vi "Logic Calculator.vi"() -> ()   [LabVIEW 2016]
panel:
  out "Loops":i32
  in  "stop":bool
  out "not(x or y)?":bool
  out "not(x and y)?":bool
  out "x or y?":bool
  out "x and y?":bool
  in  "Boolean 2":bool
  in  "Boolean":bool
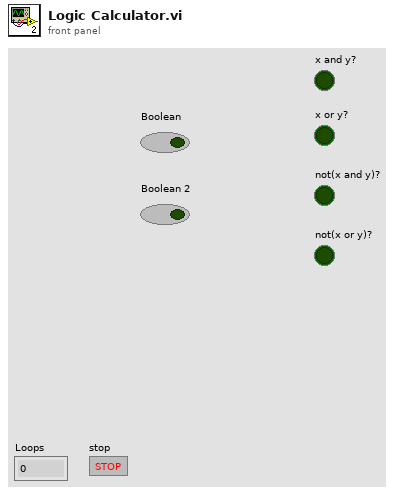
[diagram p1: front panel]
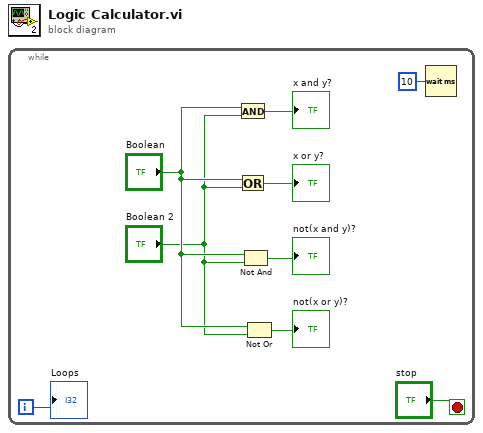
[diagram p0: block diagram]
diagram:
  n1 = while {
    i -> [w2]
    stop <- "stop" stop-if-true
    n2 = And(x="Boolean", y="Boolean 2") -> (x .and. y?=→"x and y?":bool)
    n3 = Or(x="Boolean", y="Boolean 2") -> (x .or. y?=→"x or y?":bool)
    n4 = Not And(1:"Boolean 2", 2:"Boolean") -> (0:→"not(x and y)?":bool)
    n5 = Not Or(1:"Boolean 2", 2:"Boolean") -> (0:→"not(x or y)?":bool)
    n6 = Wait (ms)(milliseconds to wait=u32 10) -> ()  [unwired: 1 out]
    "Loops" <- w2
  }
